vi "mul rtos.vi"() -> ()   [LabVIEW 2020]
uses:
  <vilib>/Analysis/Matrix/Datatypes/RealMatrix.ctl
  <vilib>/Analysis/Matrix/Numeric/Conversions/Array To Matrix - RA.vi
  <vilib>/Analysis/Matrix/Numeric/Conversions/Array To Matrix - RA2.vi
  <vilib>/Analysis/Matrix/Numeric/Multiply/Multiply - RM,RM.vi
  <vilib>/Analysis/Matrix/NI_Matrix.lvlib
panel:
  out "overall time":u32
  out "product":T1
  in  "vector size":i32=20
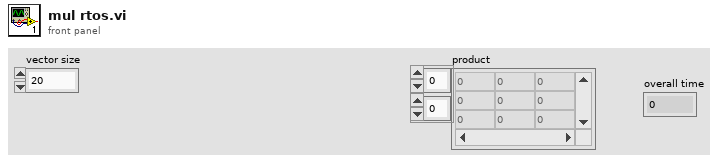
[diagram p1: front panel]
types:
  T1 = typedef "NI_Matrix.lvlib/RealMatrix.ctl" = dbl[][]
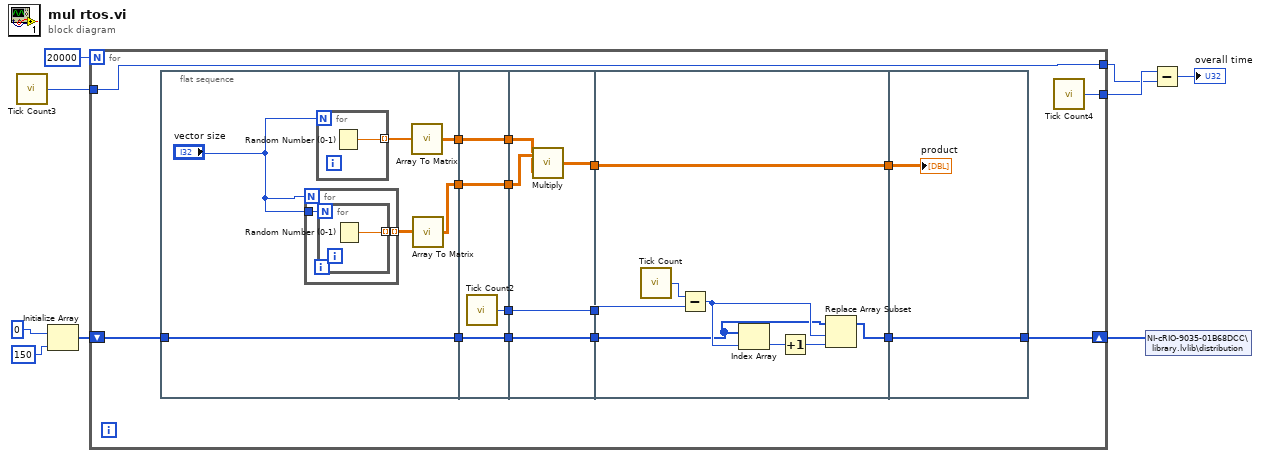
[diagram p0: block diagram]
diagram:
  n1 = call "Tick Count3"() -> ("Tick Count(uSec)"=w5:u32)
  n2 = Initialize Array(0, 150) -> (w6:i32[])
  n3 = for {
    N: 20000 -> [_]
    shift-right: [w12] -> w1
    shift-left: w6 -> [w14]
    tunnel: [w11] -> w3
    tunnel: w5 -> [w11]
    tunnel: [w10] -> w4
    n4 = flat-sequence {
      tunnel: [w30] -> w25
      tunnel: [w28] -> w19
      tunnel: [w26] -> w15
      tunnel: w14 -> [w26]
      tunnel: w25 -> [w39]
      tunnel: [w39] -> w24
      tunnel: [w38] -> w23
      tunnel: [w37] -> w20
      tunnel: w19 -> [w37]
      tunnel: [w36] -> w16
      tunnel: w15 -> [w36]
      tunnel: w24 -> [w42]
      tunnel: w23 -> [w44]
      tunnel: [w44] -> w22
      tunnel: [w41] -> w21
      tunnel: w20 -> [w43]
      tunnel: [w40] -> w17
      tunnel: w16 -> [w40]
      tunnel: w21 -> [w50]
      tunnel: w22 -> [w51]
      tunnel: [w50] -> w18
      tunnel: w17 -> [w46]
      tunnel: [w45] -> w13
      tunnel: w18 -> [w54]
      tunnel: w13 -> [w53]
      tunnel: [w53] -> w12
      frame #0 {
        n5 = for {
          N: "vector size" -> [_]
          tunnel: [w33] -> w29 mode=indexing
          tunnel: "vector size" -> [w32]
          n6 = for {
            N: w32 -> [_]
            tunnel: [w34] -> w33 mode=indexing
            n7 = Random Number (0-1)() -> (number: 0 to 1=w34:dbl)
          }
        }
        n8 = for {
          N: "vector size" -> [_]
          tunnel: [w35] -> w31 mode=indexing
          n9 = Random Number (0-1)() -> (number: 0 to 1=w35:dbl)
        }
        n10 = call-poly <vilib>:"Array To Matrix.vi"("Real 1D Array"=w31) -> ("Real Matrix (Column Vector)"=w30:T1)
        n11 = call-poly <vilib>:"Array To Matrix.vi"("Real 2D Array"=w29) -> ("Real Matrix"=w28:T1)
      }
      frame #1 {
        n12 = call "Tick Count2"() -> ("Tick Count(uSec)"=w38:u32)
      }
      frame #2 {
        n13 = call-poly <vilib>:"Multiply.vi"("Real Matrix B"=w42, "Real Matrix A"=w43) -> ("A * B"=w41:T1)
      }
      frame #3 {
        n14 = call "Tick Count"() -> ("Tick Count(uSec)"=w52:u32)
        n15 = Subtract(x=w52, y=w51) -> (x-y=w47:u32)
        n16 = Index Array(array=w46, index=w47) -> (element=w48:i32)
        n17 = Increment(x=w48) -> (x+1=w49:i32)
        n18 = Replace Array Subset(array=w46, new element=w49, index=w47) -> (w45:i32[])
      }
      frame #4 {
        "product" <- w54
      }
    }
    n19 = call "Tick Count4"() -> ("Tick Count(uSec)"=w10:u32)
  }
  n20 = shared-variable "NI-cRIO-9035-01B68DCC\\library.lvlib\\distribution"(w1) -> ()  [unwired: 1 in, 1 out]
  n21 = Subtract(x=w4, y=w3) -> (x-y=→"overall time":u32)
